vi "Init HMI.vi"(6 "Window_Title":string, 7 "Instruments":T1(array[cluster]), 8 "entrée d'erreur (pas d'erreur)":errorcluster, 10 "ce VI":refnum<vi>, 11 "Cluster en entrée":refnum<vi>) -> (0 "sortie d'erreur":errorcluster, 3 "Ref Cmd Cluster element":refnum<vi>[](array[refnum]))   [LabVIEW 2020]
uses:
  Instrument/Instrument (Default)/Class Instrument (Default).lvclass
  Commun VI/TypeDef/Commande Popup autotest/Commande element autotest.ctl
panel:
  # "膊膊"
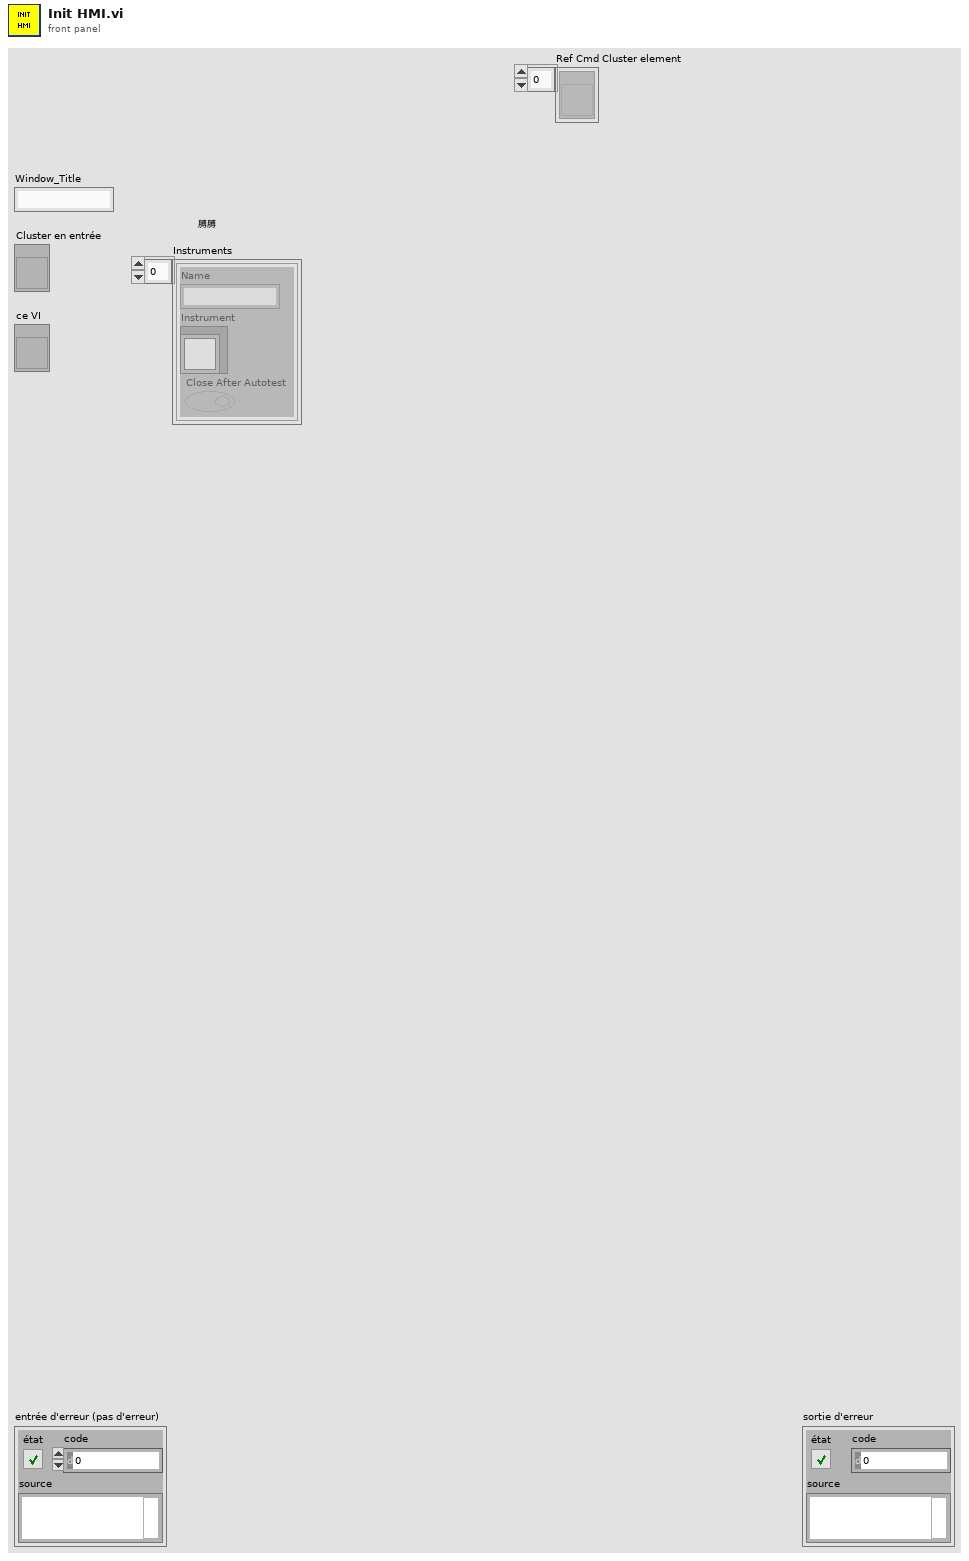
[diagram p1: front panel]
types:
  T1 = cluster{"Name":string, "Instrument":refnum<class "Class Instrument (Default).lvclass">, "Close After Autotest":bool}[]
  T2 = typedef "Commande element autotest.ctl" = cluster{"Instrument":string, "Etat":cluster{"Menu déroulant":u16}}
  T3 = cluster{"Element autotest":T2, "Element autotest 2":T2, "Element autotest 3":T2, "Element autotest 4":T2, "Element autotest 5":T2, "Element autotest 6":T2, "Element autotest 7":T2, "Element autotest 8":T2, "Element autotest 9":T2}
  T4 = typedef "LVRectTypeDef.ctl" = cluster{"Left":i16, "Top":i16, "Right":i16, "Bottom":i16}
  T5 = cluster{"[0]":T2, "[1]":T2, "[2]":T2, "[3]":T2, "[4]":T2, "[5]":T2, "[6]":T2, "[7]":T2, "[8]":T2}
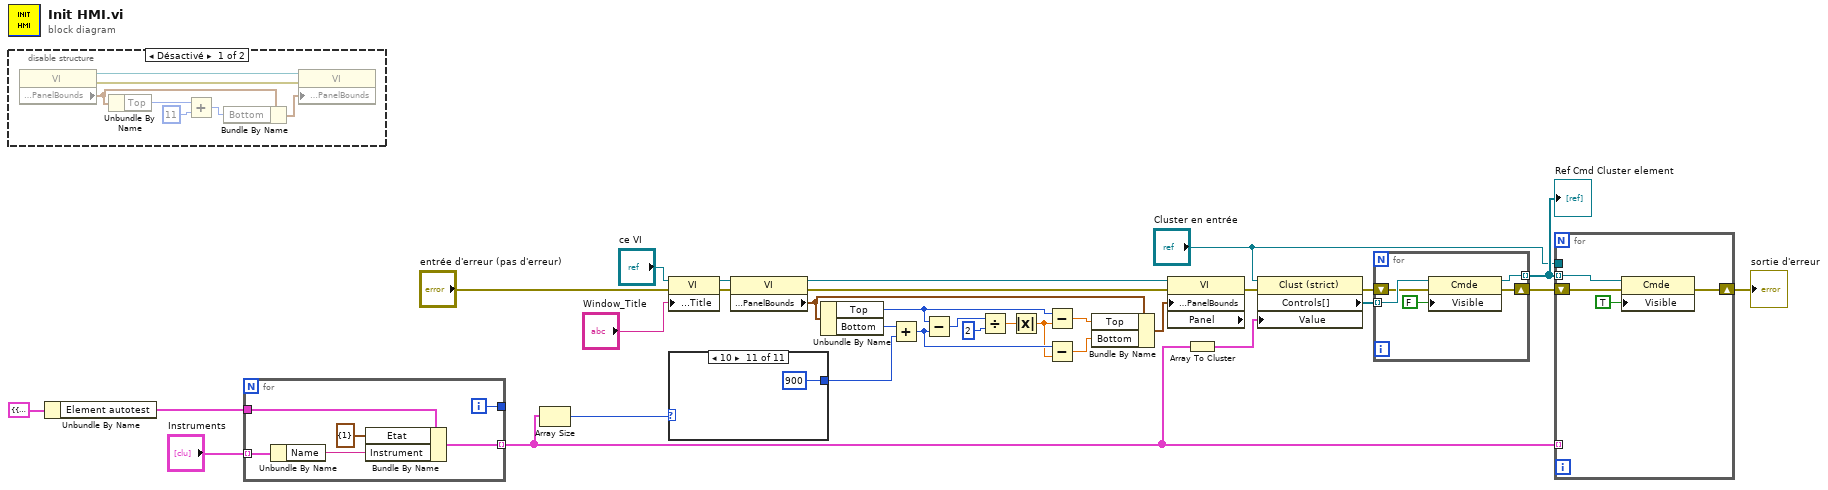
[diagram p0: block diagram]
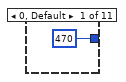
[diagram p3: hidden frame]
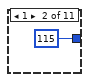
[diagram p4: hidden frame]
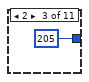
[diagram p5: hidden frame]
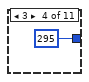
[diagram p6: hidden frame]
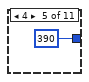
[diagram p7: hidden frame]
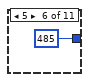
[diagram p8: hidden frame]
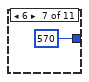
[diagram p9: hidden frame]
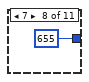
[diagram p10: hidden frame]
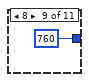
[diagram p11: hidden frame]
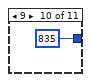
[diagram p12: hidden frame]
diagram:
  n1 = disable-structure shown="Désactivé" {
    frame Disabled {
      n2 = property class="VI"() -> (reference out=w37:refnum<vi>, error out=w39:errorcluster, "Front Panel.PanelBounds"=w38:T4)  [unwired: 2 in]
      n3 = Unbundle By Name(w38) -> ("Top"=w36:i16)
      n4 = Add(x=w36, y=i16 11) -> (x+y=w34:i16)
      n5 = Bundle By Name(cluster=w38, "Bottom"=w34) -> (w33:T4)
      n6 = property class="VI"(reference=w37, error in=w39, "Front Panel.PanelBounds"=w33) -> ()  [unwired: 2 out]
    }
    frame Enabled {
    }
  }
  n7 = Unbundle By Name(T3 {"Element autotest"={"Instrument"="", "Etat"={"Menu déroulant"=0}}, "Element autotest 2"={"Instrument"="", "Etat"={"Menu déroulant"=0}}, "Element autotest 3"={"Instrument"="", "Etat"={"Menu déroulant"=0}}, "Element autotest 4"={"Instrument"="", "Etat"={"Menu déroulant"=0}}, "Element autotest 5"={"Instrument"="", "Etat"={"Menu déroulant"=0}}, "Element autotest 6"={"Instrument"="", "Etat"={"Menu déroulant"=0}}, "Element autotest 7"={"Instrument"="", "Etat"={"Menu déroulant"=0}}, "Element autotest 8"={"Instrument"="", "Etat"={"Menu déroulant"=0}}, "Element autotest 9"={"Instrument"="", "Etat"={"Menu déroulant"=0}}} ("Element test")) -> ("Element autotest"=w22:T2)
  n8 = for {
    tunnel: "Instruments" -> [w43] mode=indexing
    tunnel: w22 -> [w45]
    tunnel: [w41] -> w20 mode=indexing
    tunnel: [w40] -> _
    i -> [w40]
    n9 = Unbundle By Name(w43) -> ("Name"=w42:string)
    n10 = Bundle By Name(cluster=w45, "Etat"=cluster{"Menu déroulant":u16} {"Menu déroulant"=1}, "Instrument"=w42) -> (w41:T2)
  }
  n11 = Array Size(array=w20) -> (size(s)=w1:i32)
  n12 = property class="VI"(reference="ce VI", error in="entrée d'erreur (pas d'erreur)", "Front Panel.Title"="Window_Title") -> (reference out=w4:refnum<vi>, error out=w5:errorcluster)
  n13 = case shown="10" w1 {
    tunnel: [i16 470 ("Bottom") i16 115 ("Bottom") i16 205 ("Bottom") i16 295 ("Bottom") i16 390 ("Bottom") i16 485 ("Bottom") i16 570 ("Bottom") i16 655 ("Bottom") i16 760 ("Bottom") i16 835 ("Bottom") i16 900 ("Bottom")] -> w15
    frame 0, Default {
    }
    frame 1 {
    }
    frame 2 {
    }
    frame 3 {
    }
    frame 4 {
    }
    frame 5 {
    }
    frame 6 {
    }
    frame 7 {
    }
    frame 8 {
    }
    frame 9 {
    }
    frame 10 {
    }
  }
  n14 = property class="VI"(reference=w4, error in=w5) -> (reference out=w6:refnum<vi>, error out=w19:errorcluster, "Front Panel.PanelBounds"=w7:T4)
  n15 = Unbundle By Name(w7) -> ("Top"=w12:i16, "Bottom"=w16:i16)
  n16 = Add(x=w16, y=w15) -> (x+y=w10:i16)
  n17 = Subtract(x=w12, y=w10) -> (x-y=w14:i16)
  n18 = Divide(x=w14, y=i16 2) -> (x/y=w13:dbl)
  n19 = Absolute Value(x=w13) -> (abs(x)=w9:dbl)
  n20 = Subtract(x=w12, y=w9) -> (x-y=w11:dbl)
  n21 = Subtract(x=w10, y=w9) -> (x-y=w8:dbl)
  n22 = Bundle By Name(cluster=w7, "Top"=w11, "Bottom"=w8) -> (w17:T4)
  n23 = property class="VI" props=["Front Panel.PanelBounds", "Panel"](reference=w6, error in=w19, "Front Panel.PanelBounds"=w17) -> (error out=w3:errorcluster)  [unwired: 2 out]
  n24 = Array To Cluster(array=w20) -> (cluster=w21:T5)
  n25 = property on="Nœud de propriété" class="Clust (strict)"(reference="Cluster en entrée", error in=w3, "Value"=w21) -> (error out=w31:errorcluster, "Controls[]"=w29:refnum<vi>[])  [unwired: 1 out]
  n26 = for {
    tunnel: w29 -> [w61] mode=indexing
    tunnel: [w59] -> w30 mode=indexing
    shift-right: [w57] -> w32
    shift-left: w31 -> [w58]
    n27 = property class="Cmde"(reference=w61, error in=w58, "Visible"=FALSE) -> (reference out=w59:refnum<vi>, error out=w57:errorcluster)
  }
  "Ref Cmd Cluster element" <- w30
  n28 = for {
    tunnel: w30 -> [w64] mode=indexing
    shift-right: [w62] -> w2
    shift-left: w32 -> [w63]
    tunnel: "Cluster en entrée" -> [_]
    tunnel: w20 -> [_] mode=indexing
    n29 = property class="Cmde"(reference=w64, error in=w63, "Visible"=TRUE) -> (error out=w62:errorcluster)  [unwired: 1 out]
  }
  "sortie d'erreur" <- w2
